vi "Write MLVCollection.vi"(8 "error in (no error)":errorcluster, 10 "MLVCollection":refnum<k24>, 11 "MongoDB-Collection in":refnum<class "MongoDB-Collection.lvclass">) -> (0 "error out":errorcluster, 3 "MongoDB-Collection out":refnum<class "MongoDB-Collection.lvclass">)   [LabVIEW 2016, in "MongoDB-Collection.lvlib" / "MongoDB-Collection.lvclass"]
uses:
  MongoDB-Collection.lvclass
  D:/Users/blume/Desktop/LV/MongoDB-Driver/MLV DLLs/MongoLabVIEW.dll
  LV/MongoDB-Driver/MLV DLLs/MongoLabVIEW.dll
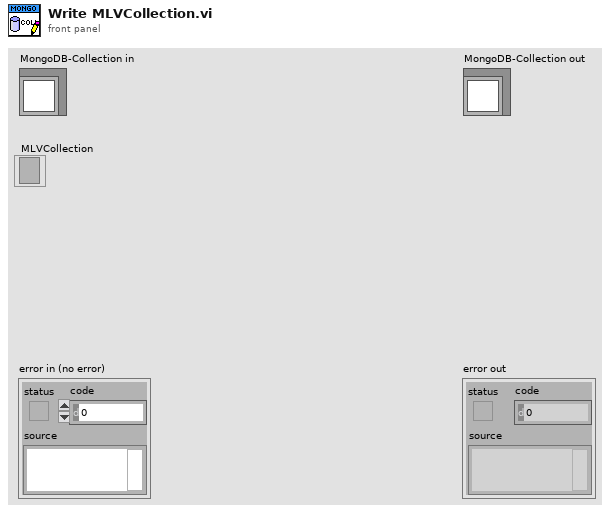
[diagram p1: front panel]
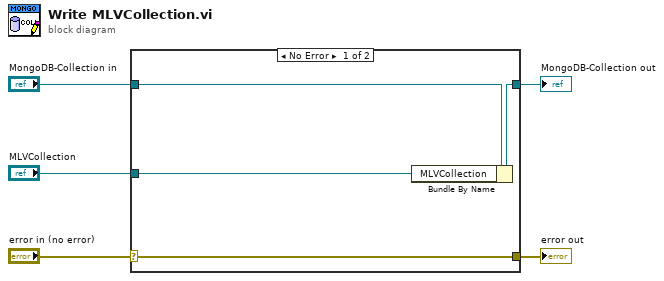
[diagram p0: block diagram]
diagram:
  n1 = case shown="No Error" "error in (no error)" {
    selector: "error in (no error)" -> [w9 w10]
    tunnel: [w9 w10] -> w4
    tunnel: [w7 w11] -> w2
    tunnel: "MongoDB-Collection in" -> [w8 w11]
    tunnel: "MLVCollection" -> [w6 _]
    frame No Error {
      n2 = Bundle By Name(cluster=w8, "MLVCollection"=w6) -> (w7:refnum<class "MongoDB-Collection.lvclass">)
    }
    frame Error {
    }
  }
  "error out" <- w4
  "MongoDB-Collection out" <- w2
